vi "Device tester (lickometer).vi"() -> ()   [LabVIEW 2015]
uses:
  Device/Typedefs/Lickometer.ctl
  Rack/Typedefs/OutputRequest refnum.ctl
  Rack/Typedefs/OutputRequest.ctl
  Rack/Typedefs/InputData cluster.ctl
  Rack/Methods/Port drivers/DigitalInput-DataCluster.ctl
  <vilib>/Platform/TimedLoop/XDataNode/timing_clust.ctl
  <vilib>/Platform/TimedLoop/XDataNode/nitl_modes.ctl
  <vilib>/Platform/TimedLoop/XDataNode/wakeup.ctl
  Rack/Methods/Rack-Init.vi
  Device/Methods/Lickometer-Init.vi
  Rack/Methods/Rack-Config.vi
  Rack/Methods/Rack-Start.vi
  Rack/Methods/Rack-Refresh.vi
  Device/Methods/Lickometer-Read.vi
  Rack/Methods/Rack-Stop.vi
  Device/Methods/Lickometer-Stop.vi
  <vilib>/platform/TimedLoop/XDataNode/XDataNode.xnode
  <vilib>/Platform/TimedLoop/XDataNode/XDNodeRunTimeDep.lvlib
panel:
  out "InputData":T1
  in  "Refresh period":i64=2
  in  "stop":bool
  out "Lick":bool
  out "#LICKS":i32
  in  "Lickometer":T3={"Settings"={"Min lick duration"=1, "Port name"="bnc_panel.p0.3", "Port index"=-1}, "Lick"=FALSE, "Debouncing"={"Semaphore"=refnum, "Lick start"=0}, "OutputRequest event ref"=refnum, "InputData reference"=refnum, "Active hi?"=FALSE}
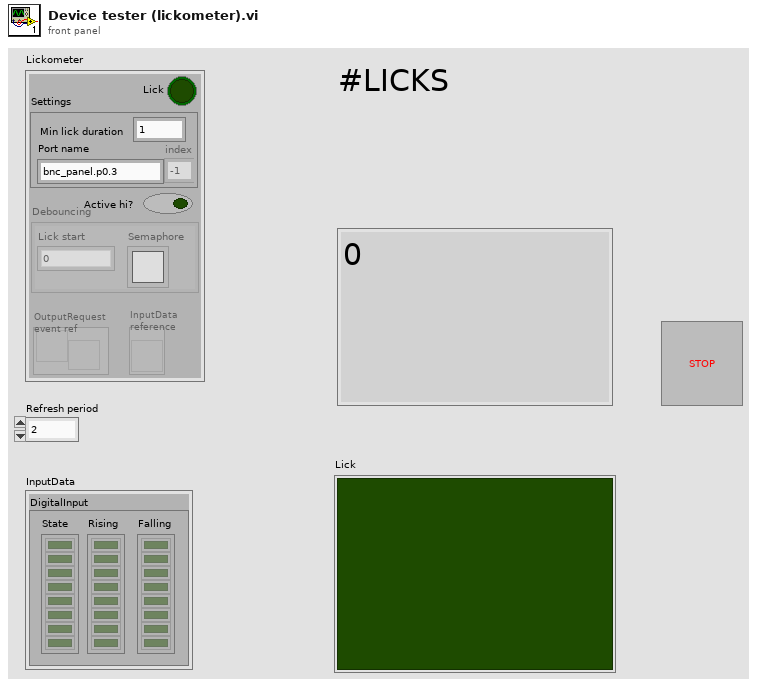
[diagram p1: front panel]
types:
  T1 = typedef "InputData cluster.ctl" = cluster{"DigitalInput":T2}
  T2 = typedef "DigitalInput-DataCluster.ctl" = cluster{"Falling":bool[], "Rising":bool[], "State":bool[]}
  T3 = typedef "Lickometer.ctl" = cluster{"Settings":cluster{"Min lick duration":u32, "Port name":string, "Port index":i32}, "Lick":bool, "Debouncing":cluster{"Semaphore":T4, "Lick start":u32}, "OutputRequest event ref":T5, "InputData reference":refnum<vi>, "Active hi?":bool}
  T4 = typedef "Semaphore RefNum" = refnum<k1>
  T5 = typedef "OutputRequest refnum.ctl" = refnum<user-event>
  T6 = typedef "Rack driver configuration cluster.ctl" = cluster{"DigitalInput":T7, "DigitalOutput":T8, "FileOutput":T9, "AnalogOutput":T10, "DataSocketOutput":T11}
  T7 = typedef "DigitalInput-Configuration.ctl" = cluster{"Lines":tag[], "Refresh period (ms)":u32}
  T8 = typedef "DigitalOutput-Configuration.ctl" = cluster{"Output Lines":tag[], "DO timestamp lines":tag[], "Timestamp lines":tag[]}
  T9 = typedef "FileOutput-Configuration.ctl" = cluster{"Logfile path":path}
  T10 = typedef "AnalogOutput-Configuration.ctl" = cluster{"Output Lines":tag[], "AO timestamp lines":tag[]}
  T11 = typedef "DataSocketOutput-Configuration.ctl" = cluster{"DataSocket URL":string}
  T12 = typedef "XDNodeRunTimeDep.lvlib/timing_clust.ctl" = cluster{"Expected End [f-1]":u64, "Actual End [f-1]":u64, "Finished Late? [f-1]":bool, "Expected End [i-1]":u64, "Actual End [i-1]":u64, "Finished Late? [i-1]":bool, "Expected Start [i]":u64, "Actual Start [i]":u64, "Expected Start [f]":u64, "Actual Start [f]":u64, "Source Name":string, "Structure Name":string, "Period":i64, "Deadline":i64, "Offset":i64, "Start":i64, "Priority":i32, "Timeout":i32, "Mode":T13, "Wakeup Reason":T14, "Error":errorcluster, "Source Type":string, "Secondary Source Type":string, "Global End Time":u64, "Global Start Time":u64, "Frame Duration":u64, "Iteration Duration":u64, "Assigned CPU":i32, "I/O Scan Engine Mode":u32}
  T13 = typedef "XDNodeRunTimeDep.lvlib/nitl_modes.ctl" = enum32{"No Change", "Process missed periods, maintain original phase", "Discard missed periods, maintain original phase", "Process missed periods, ignore original phase", "Discard missed periods, ignore original phase"}
  T14 = typedef "XDNodeRunTimeDep.lvlib/wakeup.ctl" = enum32{"Normal", "Aborted", "Asynchronous wakeup", "Timing source error", "Timed loop error", "Timeout"}
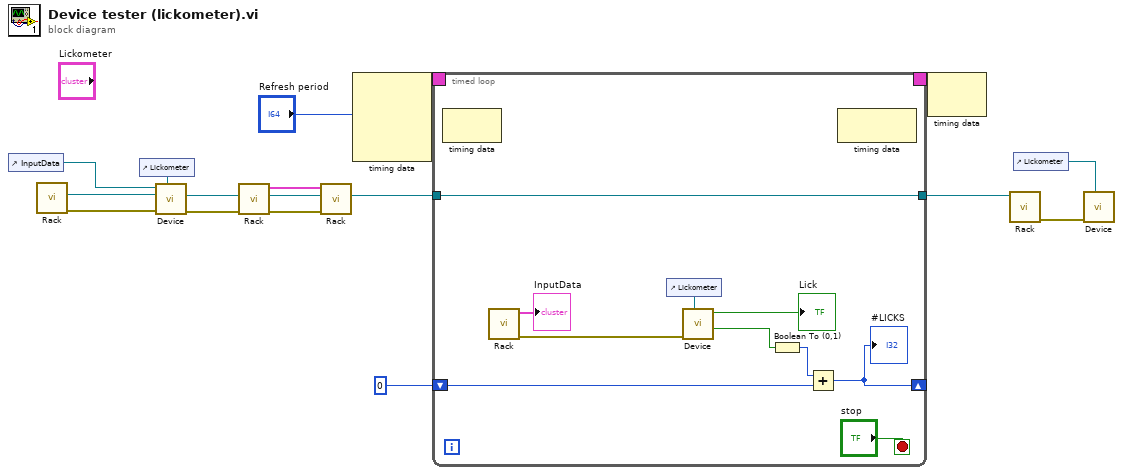
[diagram p0: block diagram]
diagram:
  n1 = control-ref of="InputData"() -> (w1:refnum<vi>)
  n2 = call-poly "Rack.vi"() -> ("error out"=w16:errorcluster, "OutputRequest\nevent ref"=w4:T5)  [unwired: 10 in]
  n3 = control-ref of="Lickometer"() -> (w15:refnum<vi>)
  n4 = call-poly "Device.vi"("Device reference"=w15, "error in (no error)"=w16, "OutputRequest event ref"=w4, "InputData reference"=w1) -> ("error out"=w14:errorcluster, "OutputRequest (dup)"=w3:T5)  [unwired: 5 in, 1 out]
  n5 = call-poly "Rack.vi"("error in (no error)"=w14) -> ("error out"=w13:errorcluster, "Configuration"=w12:T6)  [unwired: 9 in]
  n6 = call-poly "Rack.vi"("error in (no error)"=w13, "OutputRequest event ref"=w3, "Configuration"=w12) -> ("OutputRequest event ref (dup)"=w2:T5)  [unwired: 7 in, 1 out]
  n7 = node-c288("Refresh period") -> (w11:T12)  [unwired: 3 in]
  n8 = timed-loop {
    timing: w11 -> [_]
    timing-out: [_] -> w10
    tunnel: w2 -> [w25]
    tunnel: [w25] -> w9
    shift-right: [w23] -> _
    shift-left: 0 ("#LICKS") -> [w24]
    stop <- "stop" stop-if-true
    n9 = node-c288() -> ()  [unwired: 1 in, 1 out]
    n10 = call-poly "Rack.vi"() -> ("error out"=w22:errorcluster, "Data Cluster"=→"InputData":T1)  [unwired: 10 in]
    n11 = control-ref of="Lickometer"() -> (w20:refnum<vi>)
    n12 = call-poly "Device.vi"("Device reference"=w20, "error in (no error)"=w22) -> ("Lick start?"=w17:bool, "Lick?"=→"Lick":bool)  [unwired: 7 in, 1 out]
    n13 = Boolean To (0,1)(Boolean=w17) -> (0, 1=w18:i16)
    n14 = Add(x=w18, y=w24) -> (x+y=w23:i32)
    "#LICKS" <- w23
    n15 = node-c288() -> ()  [unwired: 1 in, 1 out]
  }
  n16 = node-c288(w10) -> ()  [unwired: 1 out]
  n17 = call-poly "Rack.vi"("OutputRequest channel"=w9) -> ("error out"=w6:errorcluster)  [unwired: 10 in]
  n18 = control-ref of="Lickometer"() -> (w5:refnum<vi>)
  n19 = call-poly "Device.vi"("Device reference"=w5, "error in (no error)"=w6) -> ()  [unwired: 9 in, 1 out]
